vi "Keithley 2002 ACV Config.vi"(0 "GPIB address":string="16", 1 "integration time (0:auto)":u16(ring) items=["automatic", "automatic once", "set to minimum", "set to maximum", "set aperature value", "set NPLC value"], 2 "integ. value":dbl=0.01667 format="%^.2e", 3 "range (auto:0)":u16(ring) items=["autorange", "autorange once", "set min range", "set max range", "set range value"], 4 "range value (volts)":dbl=750.0 min=0.2 max=750.0 format="%^.2e", 5 "error in":T1, 6 "coupling":bool=TRUE, 7 "resolution (4.5 digits:3)":u16(ring)=3 items=["auto resolution", "auto resolution once", "3.5 digits", "4.5 digits", "5.5 digits", "6.5 digits", "7.5 digits", "8.5 digits"], 8 "reference (off:0)":u16(ring) items=["off", "set reference value"], 9 "digital filter (off:0)":u16(ring) items=["off", "auto filter", "auto filter once", "moving filter", "repeating filter"], 10 "reference value (volts)":dbl min=-775.0 max=775.0 format="%^.2e", 11 "dig. filter count":dbl=10.0 min=1.0 max=100.0 step=1.0 format="%^.2e", 12 "AC voltage (volts:0)":u16(ring) items=["volts", "DB", "DBM"], 13 "dB reference (volts)":dbl=1.0 min=0.001 max=750.0 format="%.3f", 14 "advanced filter (off:0)":u16(ring) items=["off", "enabled"], 15 "noise tolerance (%)":dbl=5.0 min=0.0 max=100.0 step=1.0 format="%^.2e", 16 "detector (rms:0)":u16(ring) items=["RMS", "average", "low frequency RMS", "AC peak voltage", "DC negative peak spike", "DC positive peak spike"], 17 "peak window (secs)":dbl=0.1 min=0.1 max=9.9 format="%.2f", 18 "dBm ref impedance (75:1)":u16(ring)=1 items=["50 ohms", "75 ohms", "93 ohms", "132 ohms", "300 ohms", "600 ohms"]) -> (19 "error out":T1)   [LabVIEW 2020]
doc: "This VI is used to configure the settings for AC voltage measurements. The instrument can be in any mode when this VI is run. The settings will go into effect and the instrument will go into the AC voltage mode."
panel:
  # "ac\ndc"
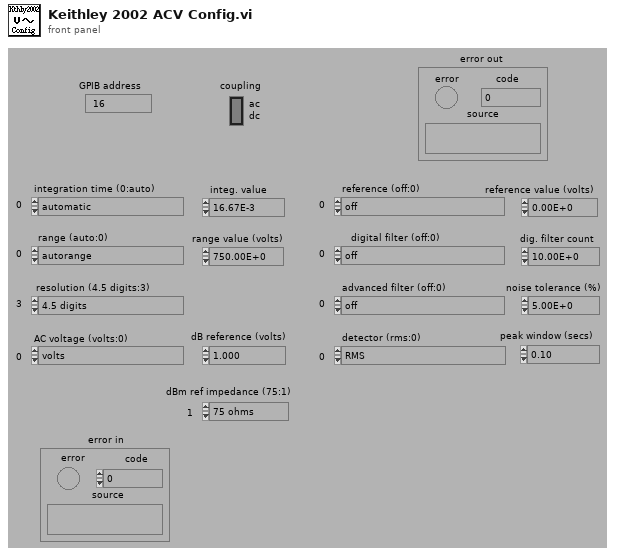
[diagram p1: front panel]
types:
  T1 = cluster{"error":bool, "code":i32, "source":string}
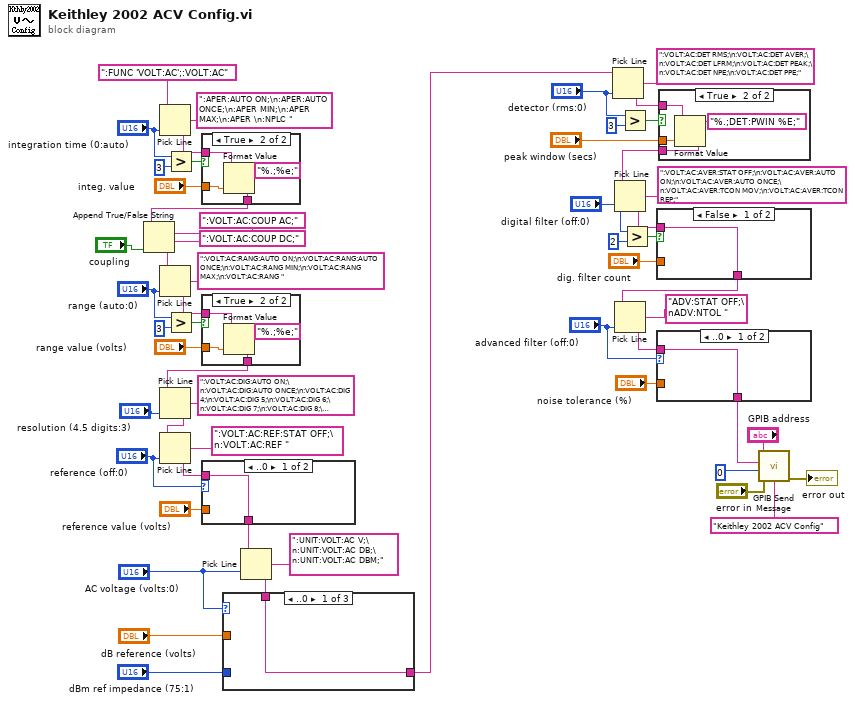
[diagram p0: block diagram]
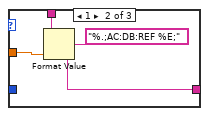
[diagram p2: hidden frame]
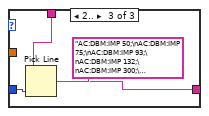
[diagram p3: hidden frame]
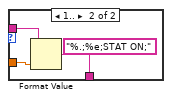
[diagram p5: hidden frame]
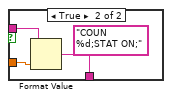
[diagram p6: hidden frame]
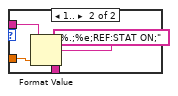
[diagram p7: hidden frame]
diagram:
  n1 = Pick Line(string ("")=":FUNC 'VOLT:AC';:VOLT:AC", multi-line string=":APER:AUTO ON;\n:APER:AUTO ONCE;\n:APER MIN;\n:APER MAX;\n:APER \n:NPLC ", line index="integration time (0:auto)") -> (output string=w51:string)
  n2 = Greater?(x="integration time (0:auto)", y=3) -> (0:w52:bool)
  n3 = Greater?(x="range (auto:0)", y=3) -> (0:w49:bool)
  n4 = case shown="True" w52 {
    tunnel: "integ. value" -> [_ w61]
    tunnel: w51 -> [w58 w60]
    tunnel: [w58 w59] -> w16
    frame False {
    }
    frame True {
      n5 = Format Value(string ("")=w60, format string="%.;%e;", value (0)=w61) -> (output string=w59:string)
    }
  }
  n6 = Append True/False String(1:"coupling", 2:":VOLT:AC:COUP DC;", 3:":VOLT:AC:COUP AC;", 4:w16) -> (0:w15:string)
  n7 = Pick Line(string ("")=w15, multi-line string=":VOLT:AC:RANG:AUTO ON;\n:VOLT:AC:RANG:AUTO ONCE;\n:VOLT:AC:RANG MIN;\n:VOLT:AC:RANG MAX;\n:VOLT:AC:RANG ", line index="range (auto:0)") -> (output string=w50:string)
  n8 = case shown="True" w49 {
    tunnel: "range value (volts)" -> [_ w66]
    tunnel: w50 -> [w63 w65]
    tunnel: [w63 w64] -> w42
    frame False {
    }
    frame True {
      n9 = Format Value(string ("")=w65, format string="%.;%e;", value (0)=w66) -> (output string=w64:string)
    }
  }
  n10 = Pick Line(string ("")=w42, multi-line string=":VOLT:AC:DIG:AUTO ON;\n:VOLT:AC:DIG:AUTO ONCE;\n:VOLT:AC:DIG 4;\n:VOLT:AC:DIG 5;\n:VOLT:AC:DIG 6;\n:VOLT:AC:DIG 7;\n:VOLT:AC:DIG 8;\n:Volt:AC:Dig 9;", line index="resolution (4.5 digits:3)") -> (output string=w38:string)
  n11 = Pick Line(string ("")=w38, multi-line string=":VOLT:AC:REF:STAT OFF;\n:VOLT:AC:REF ", line index="reference (off:0)") -> (output string=w41:string)
  n12 = case shown="..0" "reference (off:0)" {
    tunnel: "reference value (volts)" -> [_ w72]
    tunnel: w41 -> [w68 w71]
    tunnel: [w68 w69] -> w2
    frame ..0 {
    }
    frame 1.. {
      n13 = Format Value(string ("")=w71, format string="%.;%e;REF:STAT ON;", value (0)=w72) -> (output string=w69:string)
    }
  }
  n14 = Pick Line(string ("")=w2, multi-line string=":UNIT:VOLT:AC V;\n:UNIT:VOLT:AC DB;\n:UNIT:VOLT:AC DBM;", line index="AC voltage (volts:0)") -> (output string=w6:string)
  n15 = case shown="..0" "AC voltage (volts:0)" {
    tunnel: "dB reference (volts)" -> [_ w77 _]
    tunnel: [w73 w75 w80] -> w1
    tunnel: w6 -> [w73 w74 w79]
    tunnel: "dBm ref impedance (75:1)" -> [_ _ w78]
    frame ..0 {
    }
    frame 1 {
      n16 = Format Value(string ("")=w74, format string="%.;AC:DB:REF %E;", value (0)=w77) -> (output string=w75:string)
    }
    frame 2.. {
      n17 = Pick Line(string ("")=w79, multi-line string="AC:DBM:IMP 50;\nAC:DBM:IMP 75;\nAC:DBM:IMP 93;\nAC:DBM:IMP 132;\nAC:DBM:IMP 300;\nAC:DBM:IMP 600;", line index=w78) -> (output string=w80:string)
    }
  }
  n18 = Pick Line(string ("")=w1, multi-line string=":VOLT:AC:DET RMS;\n:VOLT:AC:DET AVER;\n:VOLT:AC:DET LFRM;\n:VOLT:AC:DET PEAK;\n:VOLT:AC:DET NPE;\n:VOLT:AC:DET PPE;", line index="detector (rms:0)") -> (output string=w9:string)
  n19 = Greater?(x="detector (rms:0)", y=3) -> (0:w12:bool)
  n20 = Greater?(x="digital filter (off:0)", y=2) -> (0:w32:bool)
  n21 = case shown="True" w12 {
    tunnel: "peak window (secs)" -> [_ w85]
    tunnel: w9 -> [w82 w86]
    tunnel: [w82 w83] -> w8
    frame False {
    }
    frame True {
      n22 = Format Value(string ("")=w86, format string="%.;DET:PWIN %E;", value (0)=w85) -> (output string=w83:string)
    }
  }
  n23 = Pick Line(string ("")=w8, multi-line string=":VOLT:AC:AVER:STAT OFF;\n:VOLT:AC:AVER:AUTO ON;\n:VOLT:AC:AVER:AUTO ONCE;\n:VOLT:AC:AVER:TCON MOV;\n:VOLT:AC:AVER:TCON REP;", line index="digital filter (off:0)") -> (output string=w35:string)
  n24 = case shown="False" w32 {
    tunnel: "dig. filter count" -> [_ w91]
    tunnel: w35 -> [w87 w90]
    tunnel: [w87 w89] -> w24
    frame False {
    }
    frame True {
      n25 = Format Value(string ("")=w90, format string="COUN %d;STAT ON;", value (0)=w91) -> (output string=w89:string)
    }
  }
  n26 = Pick Line(string ("")=w24, multi-line string="ADV:STAT OFF;\nADV:NTOL ", line index="advanced filter (off:0)") -> (output string=w28:string)
  n27 = case shown="..0" "advanced filter (off:0)" {
    tunnel: "noise tolerance (%)" -> [_ w96]
    tunnel: w28 -> [w92 w95]
    tunnel: [w92 w94] -> w25
    frame ..0 {
    }
    frame 1.. {
      n28 = Format Value(string ("")=w95, format string="%.;%e;STAT ON;", value (0)=w96) -> (output string=w94:string)
    }
  }
  n29 = call "GPIB Send Message.vi"("address string"="GPIB address", "write buffer"=w25, "source"="Keithley 2002 ACV Config", "write mode (set END:0)"=0, "error in"="error in") -> ("error out"=→"error out":T1)  [unwired: 2 in, 2 out]
